vi "Draw Dashed Line.vi"(4 "Direction":i32, 5 "Dynamic Origin":i32, 6 "Line Width":i32, 7 "Static Origin":i32, 8 "Dimension":i32, 9 "Color":u32(colorbox), 10 "Type":enum16{"Horizontal", "Vertical"}(ring), 11 "2D Picture in":picture) -> (3 "2D Picture out":picture)   [LabVIEW 2015]
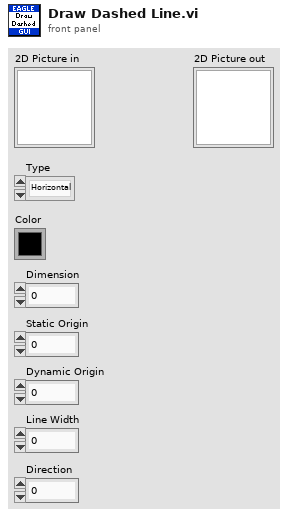
[diagram p1: front panel]
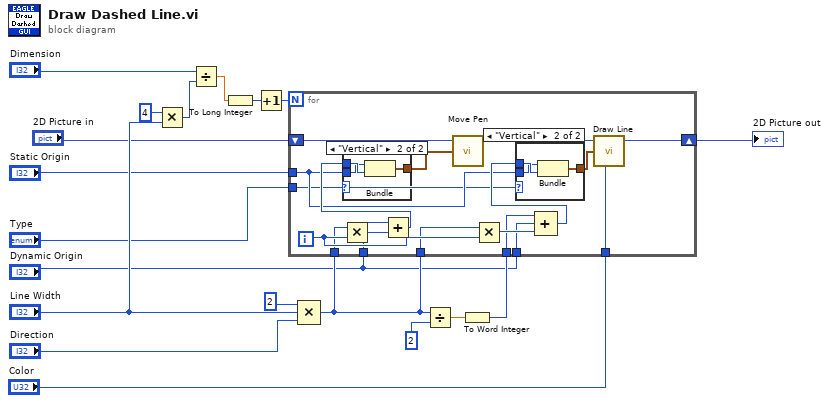
[diagram p0: block diagram]
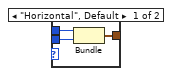
[diagram p2: hidden frame]
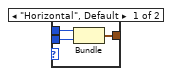
[diagram p3: hidden frame]
diagram:
  n1 = Multiply(x=4, y="Line Width") -> (x*y=w16:i32)
  n2 = Divide(x="Dimension", y=w16) -> (x/y=w17:dbl)
  n3 = To Long Integer(number=w17) -> (32bit integer=w18:i32)
  n4 = Increment(x=w18) -> (x+1=w19:i32)
  n5 = Compound Arithmetic op=MULTIPLY(2 ("x"), "Line Width", "Direction") -> (w7:i32)
  n6 = Divide(x=w7, y=2 ("x")) -> (x/y=w9:dbl)
  n7 = To Word Integer(number=w9) -> (16bit integer=w10:i16)
  n8 = for {
    N: w19 -> [_]
    shift-right: [w34] -> w13
    shift-left: "2D Picture in" -> [w37]
    tunnel: "Static Origin" -> [w23]
    tunnel: "Dynamic Origin" -> [w31]
    tunnel: "Dynamic Origin" -> [w28]
    tunnel: w7 -> [w27]
    tunnel: w7 -> [w26]
    tunnel: w10 -> [w25]
    tunnel: "Type" -> [w21]
    tunnel: "Color" -> [w20]
    i -> [w33]
    n9 = Multiply(x=w27, y=w33) -> (x*y=w32:i32)
    n10 = Add(x=w31, y=w32) -> (x+y=w30:i32)
    n11 = case shown="\"Vertical\"" w21 {
      tunnel: [w46 w49] -> w35
      tunnel: w23 -> [w45 w47]
      tunnel: w30 -> [w44 w48]
      frame "Horizontal", Default {
        n12 = Bundle(w44, "Static Origin"=w45) -> (w46:cluster{i32, "Static Origin":i32})  [unwired: 1 in]
      }
      frame "Vertical" {
        n13 = Bundle("Static Origin"=w47, w48) -> (w49:cluster{"Static Origin":i32, i32})  [unwired: 1 in]
      }
    }
    n14 = call <vilib>:"Move Pen.vi"("new position"=w35, "picture"=w37) -> ("new picture"=w36:picture)  [unwired: 3 in]
    n15 = Multiply(x=w26, y=w33) -> (x*y=w29:i32)
    n16 = Compound Arithmetic op=ADD(w25, w28, w29) -> (w24:i32)
    n17 = case shown="\"Vertical\"" w21 {
      tunnel: [w40 w43] -> w22
      tunnel: w23 -> [w39 w41]
      tunnel: w24 -> [w38 w42]
      frame "Horizontal", Default {
        n18 = Bundle(w38, "Static Origin"=w39) -> (w40:cluster{i32, "Static Origin":i32})  [unwired: 1 in]
      }
      frame "Vertical" {
        n19 = Bundle("Static Origin"=w41, w42) -> (w43:cluster{"Static Origin":i32, i32})  [unwired: 1 in]
      }
    }
    n20 = call <vilib>:"Draw Line.vi"("picture"=w36, "end point"=w22, "color(black)"=w20) -> ("new picture"=w34:picture)  [unwired: 6 in]
  }
  "2D Picture out" <- w13
